vi "DownSampleFromTime.vi"(7 "Scale(x1)":u16(ring) items=["x1"=1, "x15"=15], 8 "error in (no error)":errorcluster, 10 "Ext. Time":dbl[](array[numeric]) format="%_6g", 11 "EMG in":refnum<class "EMG.lvclass">) -> (0 "error out":errorcluster, 1 "EMG":dbl[][](array[numeric]), 2 "Ext. Time2":dbl[](array[numeric]) format="%_6g", 3 "EMG out":refnum<class "EMG.lvclass">, 4 "EMGfiltered":dbl[][](array[numeric]), 6 "ChannelNumber":i32)   [LabVIEW 2015, in "EMG.lvclass"]
uses:
  EMG.lvclass
  EMG.lvclass/EMG.ctl
  <userlib>/_OpenG.lib/array/array.llb/Conditional Auto-Indexing Tunnel (DBL)__ogtk.vi
  <vilib>/gmath/NI_Gmath.lvlib
panel:
  out "Waveform Graph":dbl[][](graph)
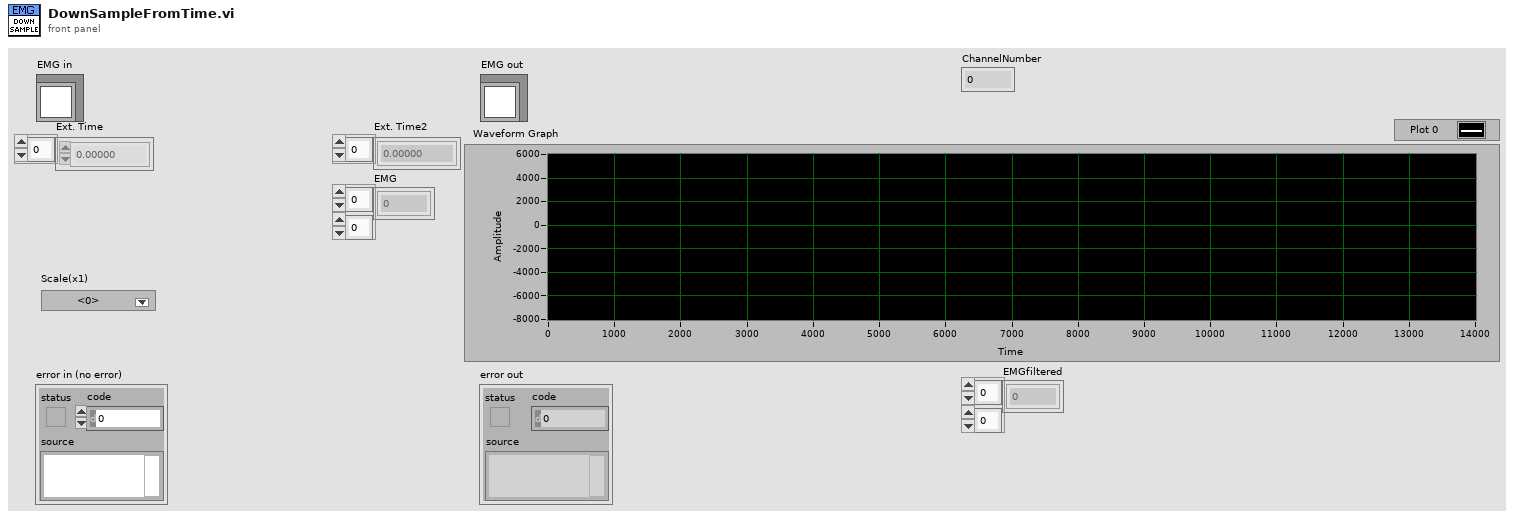
[diagram p1: front panel]
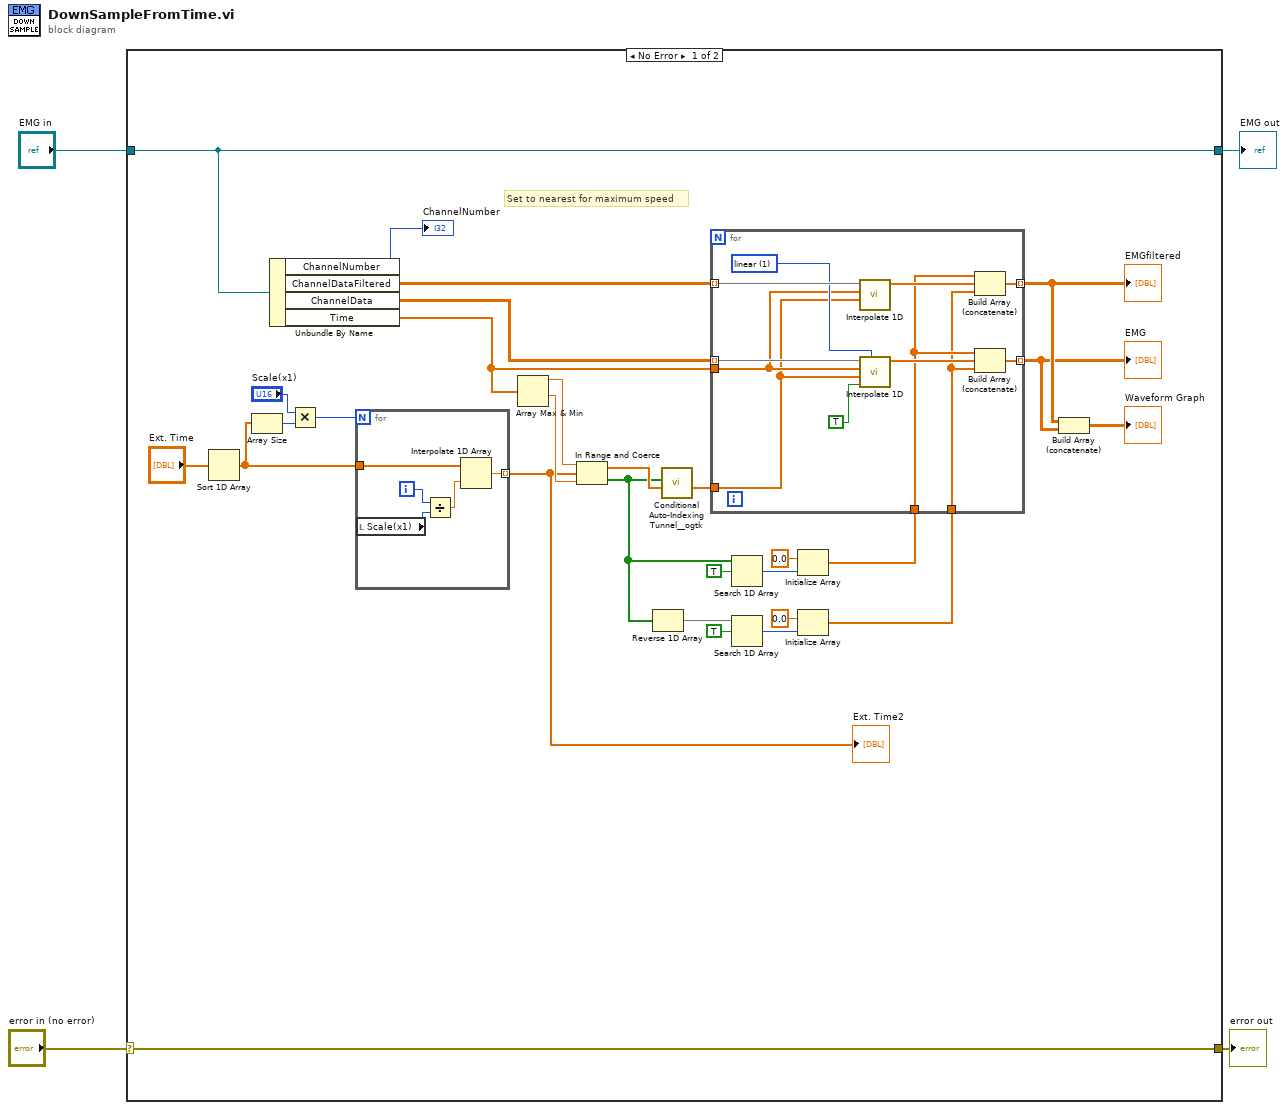
[diagram p0: block diagram]
diagram:
  n1 = case shown="No Error" "error in (no error)" {
    selector: "error in (no error)" -> [w33 w52]
    tunnel: [w33 w52] -> w3
    tunnel: [w32 w51] -> w1
    tunnel: "EMG in" -> [w32 w51]
    frame No Error {
      # "Set to nearest for maximum speed"
      n2 = Sort 1D Array(array="Ext. Time") -> (sorted array=w16:dbl[])
      n3 = Array Size(array=w16) -> (size(s)=w15:i32)
      n4 = Unbundle By Name(w32) -> ("ChannelNumber"=→"ChannelNumber":i32, "ChannelDataFiltered"=w7:dbl[][], "ChannelData"=w6:dbl[][], "Time"=w9:dbl[])
      n5 = Multiply(x="Scale(x1)", y=w15) -> (x*y=w5:i32)
      n6 = for {
        N: w5 -> [_]
        tunnel: w16 -> [w38]
        tunnel: [w37] -> w17 mode=indexing
        i -> [w35]
        n7 = local read "Scale(x1)"() -> (w34:u16)
        n8 = Divide(x=w35, y=w34) -> (x/y=w36:dbl)
        n9 = Interpolate 1D Array(1:w36, 2:w38) -> (0:w37:dbl)
      }
      "Ext. Time2" <- w17
      n10 = Array Max & Min(array=w9) -> (max value=w30:dbl, min value=w31:dbl)  [unwired: 2 out]
      n11 = In Range and Coerce(upper limit=w30, x=w17, lower limit=w31) -> (coerced(x)=w22:dbl[], In Range?=w21:bool[])
      n12 = Reverse 1D Array(array=w21) -> (reversed array=w25:bool[])
      n13 = call-poly <userlib>:"Conditional Auto-Indexing Tunnel__ogtk.vi"("Array in"=w22, "Elements to keep"=w21) -> ("Filtered Array out"=w8:dbl[])  [unwired: 5 in]
      n14 = Search 1D Array(1D array=w21, element=TRUE) -> (index of element=w26:i32)  [unwired: 1 in]
      n15 = Search 1D Array(1D array=w25, element=TRUE) -> (index of element=w23:i32)  [unwired: 1 in]
      n16 = Initialize Array(0.0 ("element"), w26) -> (w20:dbl[])
      n17 = Initialize Array(0.0 ("element"), w23) -> (w19:dbl[])
      n18 = for {
        tunnel: w6 -> [w50] mode=indexing
        tunnel: w9 -> [w40]
        tunnel: w8 -> [w39]
        tunnel: w20 -> [w44]
        tunnel: w19 -> [w43]
        tunnel: [w48] -> w12 mode=indexing
        tunnel: w7 -> [w47] mode=indexing
        tunnel: [w42] -> w13 mode=indexing
        w41 = 1 items=["nearest", "linear", "spline", "cubic Hermite", "Lagrange"] ("method")
        n19 = call <vilib>:"Interpolate 1D.vi"("xi"=w39, "X"=w40, "Y"=w47) -> ("yi"=w45:dbl[])  [unwired: 6 in, 2 out]
        n20 = call <vilib>:"Interpolate 1D.vi"("method"=w41, "X is monotonic"=TRUE, "xi"=w39, "X"=w40, "Y"=w50) -> ("yi"=w49:dbl[])  [unwired: 4 in, 2 out]
        n21 = Build Array (concatenate)(w44, w45, w43) -> (w42:dbl[])
        n22 = Build Array (concatenate)(w44, w49, w43) -> (w48:dbl[])
      }
      "EMG" <- w12
      "EMGfiltered" <- w13
      n23 = Build Array (concatenate)(w13, w12) -> (→"Waveform Graph":dbl[][])
    }
    frame Error {
    }
  }
  "error out" <- w3
  "EMG out" <- w1
